vi "test.Create.Time.vi"() -> (3 "Passed":bool)   [LabVIEW 2020]
uses:
  Time/Time.Parameters.ctl
  Time/Time.lvclass
panel:
  out "Boolean":bool
  in  "Time.Parameters":T1
  out "x = y?":bool[](array[boolean])
  out "Python.Bytes.Out":u8[](array[numeric]) format="%.0x"
  out "LabVIEW.Bytes.Out":u8[](array[numeric]) format="%.0x"
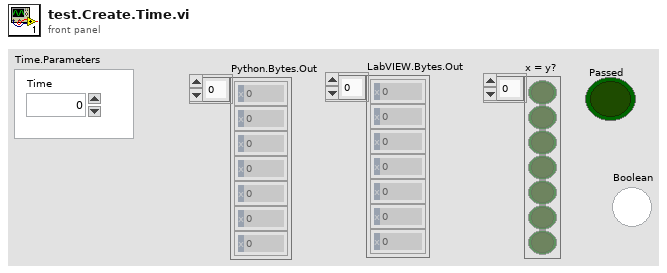
[diagram p1: front panel]
types:
  T1 = typedef "Time.lvclass/Time.Parameters.ctl" = cluster{"Time":u32}
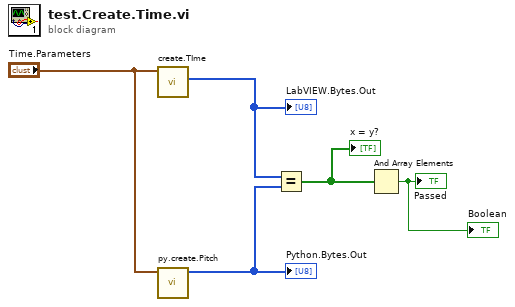
[diagram p0: block diagram]
diagram:
  n1 = call "create.TIme.vi"("Time.Parameters"="Time.Parameters") -> ("Bytes.Out"=w5:u8[])  [unwired: 8 in, 2 out]
  "LabVIEW.Bytes.Out" <- w5
  n2 = call "py.create.Pitch.vi"("Parameters"="Time.Parameters") -> ("bytes"=w4:u8[])  [unwired: 9 in, 1 out]
  "Python.Bytes.Out" <- w4
  n3 = Equal?(x=w5, y=w4) -> (x = y?=w3:bool[])
  "x = y?" <- w3
  n4 = And Array Elements(Boolean array=w3) -> (logical AND=→"Passed" →"Boolean":bool)
